vi "Desktop Main.vi"() -> ()   [LabVIEW 2021]
doc: "Demonstrates how to use User Datagram Protocol (UDP) to send data to the myRIO target."
panel:
  out "Tank":dbl(slide) scale=0.0..10.0
  out "error out":errorcluster
  in  "Stop":bool
  in  "Target IP Address":string="172.22.11.2"
  # "Overview: Demonstrates how to use User Datagram Protocol (UDP) to send data to the myRIO target.\nInstructions:\n1. Verify the value of Target IP Address. If it is incorrect, specify the correct value.\n2. (Optional) To broadcast data to several myRIO targets without specifying their IP addresses, set the value of Target IP Address to one of the following values:\n    - 255.255.255.255\n    - 192.168.1.255, if your IP address is in the form 192.168.1.x.\n3. Run this VI.\n4. Open RT Main.vi and follow its front panel instructions.\n5. Click Stop to stop this VI."
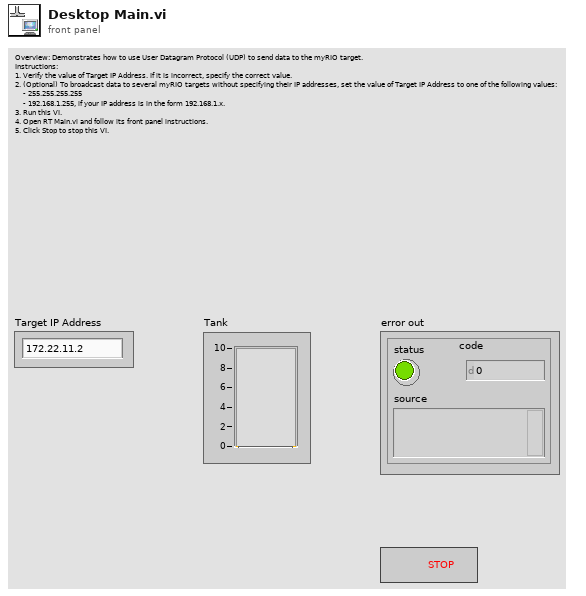
[diagram p1: front panel]
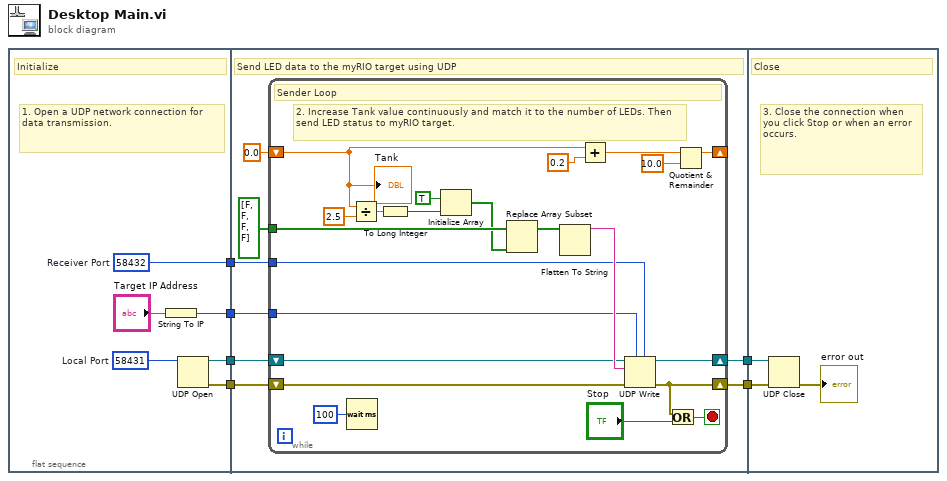
[diagram p0: block diagram]
diagram:
  n1 = flat-sequence {
    tunnel: [w12] -> w4
    tunnel: [w11] -> w3
    tunnel: [w8] -> w2
    tunnel: [w7] -> w1
    tunnel: [w20] -> w6
    tunnel: [w19] -> w5
    tunnel: w4 -> [w18]
    tunnel: w3 -> [w17]
    tunnel: w2 -> [w16]
    tunnel: w1 -> [w14]
    tunnel: w6 -> [w44]
    tunnel: w5 -> [w45]
    frame #0 {
      w7 = u16 58432  # Receiver Port
      w10 = u16 58431  # Local Port
      # "1. Open a UDP network connection for data transmission."
      # "Initialize"
      n2 = String To IP(1:"Target IP Address") -> (0:w8:u32)
      n3 = UDP Open(11:w10) -> (port=w12:refnum<k16>, 0:w11:errorcluster)  [unwired: 4 in, 1 out]
    }
    frame #1 {
      # "Send LED data to the myRIO target using UDP"
      n4 = while {
        shift-right: [w33] -> w20
        shift-left: w17 -> [w26]
        shift-right: [w38] -> w19
        shift-left: w18 -> [w27]
        tunnel: w16 -> [w32]
        shift-right: [w28] -> _
        shift-left: 0.0 ("y") -> [w36]
        tunnel: w14 -> [w31]
        tunnel: bool[] [FALSE, FALSE, FALSE, FALSE] -> [w23]
        stop <- w42 stop-if-true
        # "2. Increase Tank value continuously and match it to the number of LEDs. Then send LED status to myRIO target."
        # "Sender Loop"
        n5 = Wait (ms)(milliseconds to wait=u32 100) -> ()  [unwired: 1 out]
        n6 = Divide(x=w36, y=2.5) -> (x/y=w40:dbl)
        n7 = To Long Integer(number=w40) -> (32bit integer=w24:i32)
        n8 = Initialize Array(TRUE, w24) -> (w21:bool[])
        n9 = Replace Array Subset(array=w23, new element=w21) -> (w22:bool[])  [unwired: 1 in]
        n10 = Flatten To String(anything=w22) -> (data string=w39:string)  [unwired: 3 in, 2 out]
        n11 = Add(x=w36, y=0.2) -> (x+y=w29:dbl)
        n12 = UDP Write(address=w32, port or service name=w31, connection ID=w27, data in=w39, 8:w26) -> (error out=w33:errorcluster, 3:w38:refnum<k16>)  [unwired: 1 in]
        n13 = Or(x=w33, y="Stop") -> (x .or. y?=w42:bool)
        n14 = Quotient & Remainder(x=w29, y=10.0) -> (x-y*floor(x/y)=w28:dbl)  [unwired: 1 out]
        "Tank" <- w36
      }
    }
    frame #2 {
      # "3. Close the connection when you click Stop or when an error occurs."
      # "Close"
      n15 = UDP Close(connection ID=w45, 8:w44) -> (error out=→"error out":errorcluster)  [unwired: 1 out]
    }
  }
